vi "ReleaseQueueTCPIP.vi"(8 "error in (no error)":errorcluster, 11 "Server in":refnum<class "Server.lvclass">) -> (0 "error out":errorcluster, 3 "Server out":refnum<class "Server.lvclass">)   [LabVIEW 2018, in "Server.lvclass"]
uses:
  Server.lvclass
  Server.lvclass/Server.ctl
panel:
  out "remaining elements":T1(array[cluster])
  out "queue name":string
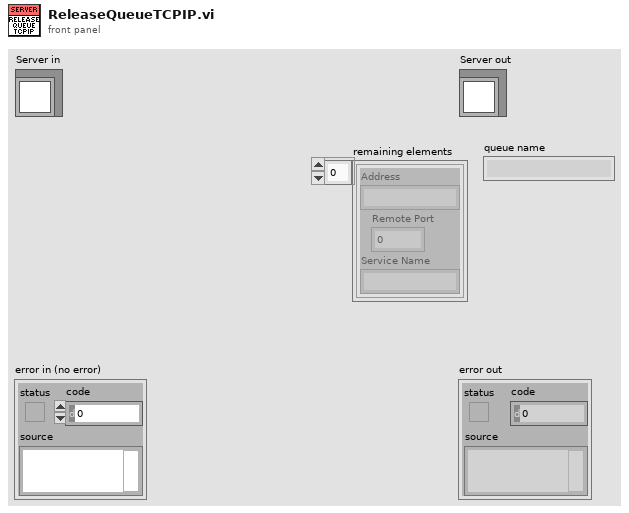
[diagram p1: front panel]
types:
  T1 = cluster{"Address":string, "Remote Port":u32, "Service Name":string}[]
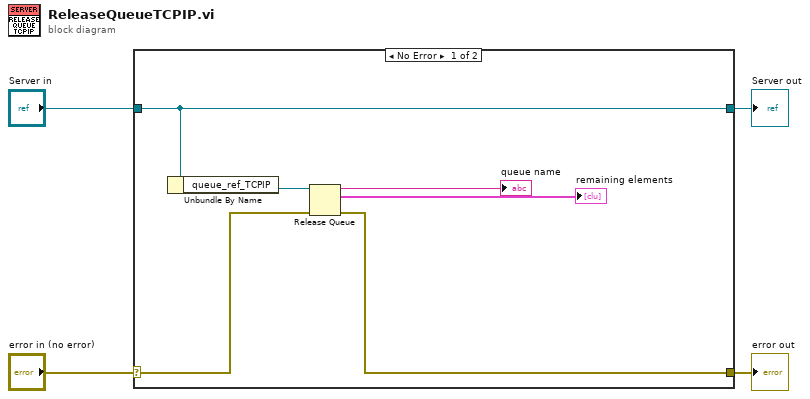
[diagram p0: block diagram]
diagram:
  n1 = case shown="No Error" "error in (no error)" {
    selector: "error in (no error)" -> [w8 w12]
    tunnel: [w7 w12] -> w3
    tunnel: [w10 w11] -> w1
    tunnel: "Server in" -> [w10 w11]
    frame No Error {
      n2 = Unbundle By Name(w10) -> ("queue_ref_TCPIP"=w9:refnum<queue>)
      n3 = Release Queue(queue=w9, error in (no error)=w8) -> (queue name=→"queue name":string, remaining elements=→"remaining elements":T1, error out=w7:errorcluster)  [unwired: 1 in]
    }
    frame Error {
    }
  }
  "error out" <- w3
  "Server out" <- w1
